vi "Get Result.vi"(8 "error in (no error)":errorcluster, 11 "Visa instrument in":refnum<class "Visa instrument.lvclass">) -> (0 "error out":errorcluster, 2 "Mag Lab Result.lvclass":refnum<class "Mag Lab Result.lvclass">, 3 "Visa instrument out":refnum<class "Visa instrument.lvclass">)   [LabVIEW 2015, in "Visa instrument.lvclass"]
uses:
  Visa instrument.lvclass
  Mag Lab Result/Mag Lab Result.lvclass
  Mag Lab Hardware.lvclass/Mag Lab Hardware.ctl
  Mag Lab Root/Mag Lab Root.lvclass/Mag Lab Root.ctl
  Mag Lab Error Handler/Mag Lab Error Handler.lvclass
  Mag Lab Hardware.lvclass
  Mag Lab Root/Mag Lab Root.lvclass
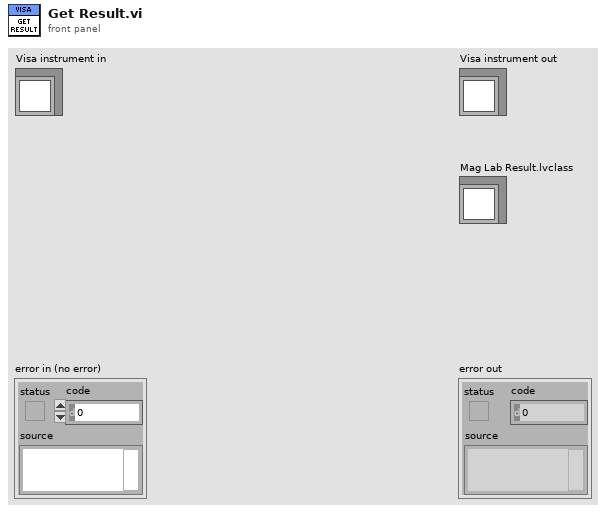
[diagram p1: front panel]
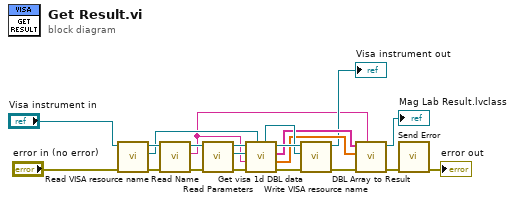
[diagram p0: block diagram]
diagram:
  n1 = call "Read VISA resource name.vi"("error in (no error)"="error in (no error)", "Mag Lab Hardware in"="Visa instrument in") -> ("error out"=w19:errorcluster, "VISA resource name"=w2:refnum<visa-resource-name>, "Mag Lab Hardware out"=w20:refnum<class "Visa instrument.lvclass">)  [unwired: 7 in]
  n2 = call "Read Name.vi"("error in (no error)"=w19, "Mag Lab Root in"=w20) -> ("error out"=w17:errorcluster, "Name"=w1:string, "Mag Lab Root out"=w16:refnum<class "Visa instrument.lvclass">)  [unwired: 7 in]
  n3 = call-dynamic "Read Parameters.vi"("error in (no error)"=w17, "Mag Lab Root in"=w16) -> ("error out"=w6:errorcluster, "Mag Lab Parameters.lvclass"=w7:refnum<class "Mag Lab Parameters.lvclass">, "Mag Lab Root out"=w15:refnum<class "Visa instrument.lvclass">)  [unwired: 7 in]
  n4 = call-dynamic "Get visa 1d DBL data.vi"("VISA resource name"=w2, "error in (no error)"=w6, "Name"=w1, "Mag Lab Parameters in"=w7, "Visa instrument in"=w15) -> ("error out"=w13:errorcluster, "Channel data"=w10:dbl[], "Channel names"=w11:string[], "Visa instrument out"=w14:refnum<class "Visa instrument.lvclass">, "VISA resource name out"=w12:refnum<visa-resource-name>)  [unwired: 2 in]
  n5 = call "Write VISA resource name.vi"("error in (no error)"=w13, "VISA resource name"=w12, "Mag Lab Hardware in"=w14) -> ("error out"=w18:errorcluster, "Mag Lab Hardware out"=→"Visa instrument out":refnum<class "Visa instrument.lvclass">)  [unwired: 7 in]
  n6 = call "DBL Array to Result.vi"("Result name"=w1, "error in (no error)"=w18, "Data"=w10, "Channel Names"=w11) -> ("error out"=w4:errorcluster, "Mag Lab Result out"=→"Mag Lab Result.lvclass":refnum<class "Mag Lab Result.lvclass">)  [unwired: 6 in]
  n7 = call "Send Error.vi"("error in (no error)"=w4) -> ("error out"=→"error out":errorcluster)  [unwired: 9 in, 1 out]
